vi "Z_switch_VCH.vi"(10 "Z":T1={"Z_HSw"=1, "Z_HSetState"=enum."on (closed)", "Z_ASetState"=enum."on (closed)", "Z_DSetState"=enum."on (closed)"}, 11 "Z_LSw (2-auto)":u32=2) -> (2 "Z_SetState":T2=enum."on (closed)", 3 "Z_Source":T3=enum."local disabled")   [LabVIEW 2019, in "Valves.lvlib"]
uses:
  Valves.lvlib
  ctl/Z_State_VCH.ctl
  Heating/ctl/Z_source.ctl
  ctl/Z_control_VCH.ctl
  Heating/Heating.lvlib
panel:
  # "Z_Source(Z1) – источник управления\nZ_Source – источник управления:\n     0 – initialize (Инициализация)\n     1 – local disabled (Выведен из работы по месту)\n     2 – local hand (Ручной местный)\n     3 – hand (Ручной контроллера)\n     4 – auto (Автомат контроллера)\n     5 – dist (Дистанционный)\nZ_SetState_VCH(Z2) заданное состояние автомата механизма:\n     1 – alarm (авария)\n     2 – disabled (выведен из работы)\n     4 – stop (стоп - готов к работе)\n     5 – reserv (резерв)\n     9 – check (проверка работоспособности)\n     12 – on (включен)\nСостояние\nZ_State_VCH(Z3) состояние автомата механизма:\n     0 – init (инициализация)\n     1 – alarm (авария)\n     2 – disabled (выведен из работы)\n     3 – not ready (не готов к работе)\n     4 – closed ready (закрыт - готов к работе)\n     5 – reserv (резерв)\n     9 – check (проверка работоспособности)\n     11 – open (открыт)\n     12 – on (закрыт)"
  # "Входы\nZ_LSw – переключатель р/а. 1 приоритет\n     0 – откл\n     1 – ручной (местный)\n     2 – автомат\nZ_HSw – источник управления из меню. 2 приоритет\n     0 – ручной контроллера\n     1 – автомат контроллера\n     2 – дистационный\nZ_HSetState – заданное состояние в меню или на панели\nZ_ASetState – заданное состояние от вышестоящего алгоритма\nZ_DSetState – заданное состояние дистанционно\n     1 – alarm (авария)\n     2 – disabled (выведен из работы)\n     4 – stop (стоп - готов к работе)\n     5 – reserv (резерв)\n     9 – check (проверка работоспособности)\n     12 – on (включен)\n     13... -> 3 – стоп"
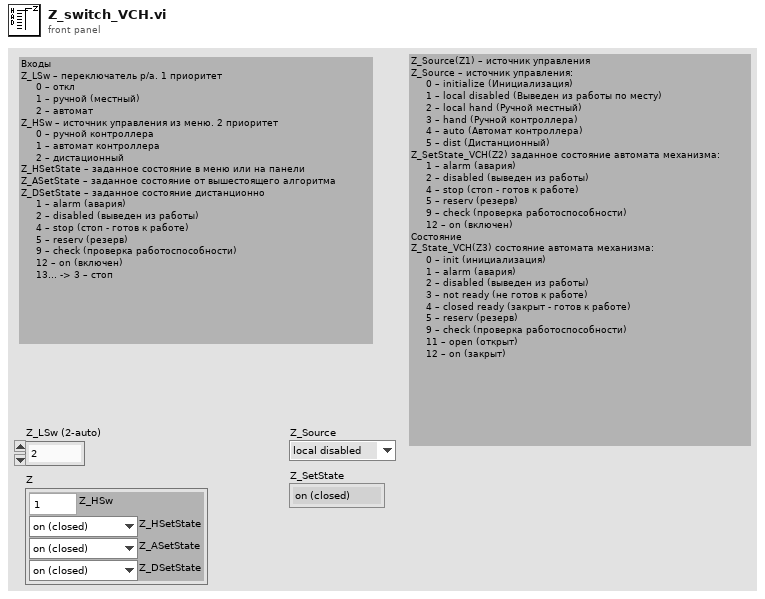
[diagram p1: front panel]
types:
  T1 = typedef "Valves.lvlib/Z_control_VCH.ctl" = cluster{"Z_HSw":u8, "Z_HSetState":T2, "Z_ASetState":T2, "Z_DSetState":T2}
  T2 = typedef "Valves.lvlib/Z_State_VCH.ctl" = enum8{"initialization", "alarm", "disabled", "not ready", "closed ready", "reserv", "reserv1", "reserv2", "reserv3", "check", "on min", "open", "on (closed)"}
  T3 = typedef "Heating.lvlib/Z_source.ctl" = enum8{"initialize", "local disabled", "local hand", "hand", "auto", "dist"}
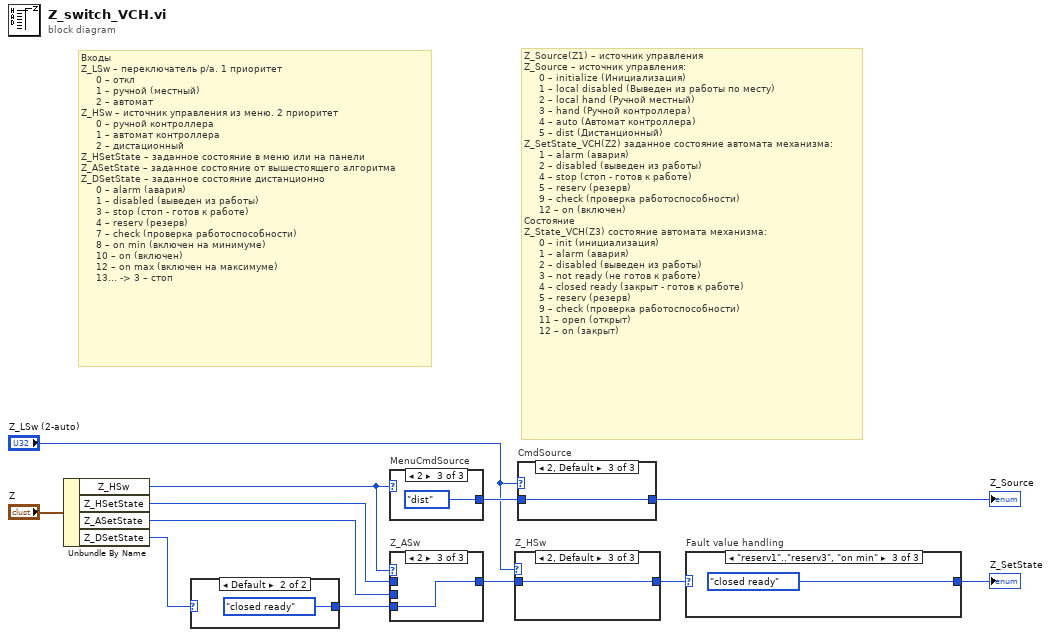
[diagram p0: block diagram]
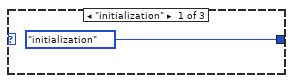
[diagram p2: hidden frame]
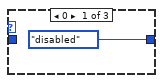
[diagram p7: hidden frame]
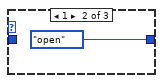
[diagram p8: hidden frame]
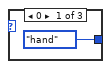
[diagram p9: hidden frame]
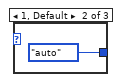
[diagram p10: hidden frame]
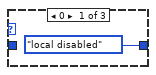
[diagram p11: hidden frame]
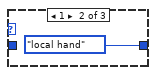
[diagram p12: hidden frame]
diagram:
  # "Входы\nZ_LSw – переключатель р/а. 1 приоритет\n     0 – откл\n     1 – ручной (местный)\n     2 – автомат\nZ_HSw – источник управления из меню. 2 приоритет\n     0 – ручной контроллера\n     1 – автомат контроллера\n     2 – дистационный\nZ_HSetState – заданное состояние в меню или на панели\nZ_ASetState – заданное состояние от вышестоящего алгоритма\nZ_DSetState – заданное состояние дистанционно\n     0 – alarm (авария)\n     1 – disabled (выведен из работы)\n     3 – stop (стоп - готов к работе)\n     4 – reserv (резерв)\n     7 – check (проверка работоспособности)\n     8 – on min (включен на минимуме)\n     10 – on (включен)\n     12 – on max (включен на максимуме)\n     13... -> 3 – стоп"
  # "Z_Source(Z1) – источник управления\nZ_Source – источник управления:\n     0 – initialize (Инициализация)\n     1 – local disabled (Выведен из работы по месту)\n     2 – local hand (Ручной местный)\n     3 – hand (Ручной контроллера)\n     4 – auto (Автомат контроллера)\n     5 – dist (Дистанционный)\nZ_SetState_VCH(Z2) заданное состояние автомата механизма:\n     1 – alarm (авария)\n     2 – disabled (выведен из работы)\n     4 – stop (стоп - готов к работе)\n     5 – reserv (резерв)\n     9 – check (проверка работоспособности)\n     12 – on (включен)\nСостояние\nZ_State_VCH(Z3) состояние автомата механизма:\n     0 – init (инициализация)\n     1 – alarm (авария)\n     2 – disabled (выведен из работы)\n     3 – not ready (не готов к работе)\n     4 – closed ready (закрыт - готов к работе)\n     5 – reserv (резерв)\n     9 – check (проверка работоспособности)\n     11 – open (открыт)\n     12 – on (закрыт)"
  n1 = Unbundle By Name("Z") -> ("Z_HSw"=w4:u8, "Z_HSetState"=w3:T2, "Z_ASetState"=w2:T2, "Z_DSetState"=w1:T2)
  n2 = case shown="Default" w1 {
    selector: w1 -> [w13 _]
    tunnel: [w13 Z_State_VCH."closed ready" ("X5(DistSetSate) 2")] -> w8
    frame "alarm".."on (closed)" {
    }
    frame Default {
    }
  }
  n3 = case "MenuCmdSource" shown="2" w4 {
    tunnel: [Z_source."hand" ("Z1(CmdSource) 3") Z_source."auto" ("Z1(CmdSource) 3") Z_source."dist" ("Z1(CmdSource) 3")] -> w12
    frame 0 {
    }
    frame 1, Default {
    }
    frame 2 {
    }
  }
  n4 = case "Z_ASw" shown="2" w4 {
    tunnel: [w18 w19 w20] -> w10
    tunnel: w3 -> [w18 _ _]
    tunnel: w8 -> [_ _ w20]
    tunnel: w2 -> [_ w19 _]
    frame 0 {
    }
    frame 1, Default {
    }
    frame 2 {
    }
  }
  n5 = case "Z_HSw" shown="2, Default" "Z_LSw (2-auto)" {
    tunnel: [Z_State_VCH."disabled" ("X5(DistSetSate) 2") Z_State_VCH."open" ("X5(DistSetSate) 2") w23] -> w9
    tunnel: w10 -> [_ _ w23]
    frame 0 {
    }
    frame 1 {
    }
    frame 2, Default {
    }
  }
  n6 = case "CmdSource" shown="2, Default" "Z_LSw (2-auto)" {
    tunnel: [Z_source."local disabled" ("Z1(CmdSource) 3") Z_source."local hand" ("Z1(CmdSource) 3") w26] -> w6
    tunnel: w12 -> [_ _ w26]
    frame 0 {
    }
    frame 1 {
    }
    frame 2, Default {
    }
  }
  "Z_Source" <- w6
  n7 = case "Fault value handling" shown="\"reserv1\"..\"reserv3\", \"on min\"" w9 {
    selector: w9 -> [_ w28 _]
    tunnel: [Z_State_VCH."initialization" ("X5(DistSetSate) 2") w28 Z_State_VCH."closed ready" ("X5(DistSetSate) 2")] -> w7
    frame "initialization" {
    }
    frame "alarm".."reserv", "check", "open", "on (closed)", Default {
    }
    frame "reserv1".."reserv3", "on min" {
    }
  }
  "Z_SetState" <- w7
